vi "RIB Req - MCCB AUX Status.vi"(0 "Limits File Path":path, 5 "Results File Path":path, 11 "error in":errorcluster) -> (4 "Results Data Array":string[][](array[string]), 15 "error out":errorcluster)   [LabVIEW 2024]
doc: "Template test"
uses:
  <vilib>/addons/_JKI Toolkits/State Machine/_JKI_lib_State_Machine.llb/Select State(s)_err__jki_lib_state_machine.vi
  <vilib>/addons/_JKI Toolkits/State Machine/_JKI_lib_State_Machine.llb/Periodic Trigger__ogtk__JKI-SM__jki_lib_state_machine.vi
  <userlib>/_OpenG.lib/file/file.llb/Strip Path Extension - String__ogtk.vi
  <vilib>/Utility/file.llb/Read Delimited Spreadsheet (string).vi
  <userlib>/_OpenG.lib/file/file.llb/openg_file.lvlib
  <userlib>/_OpenG.lib/appcontrol/appcontrol.llb/openg_application_control.lvlib
  <userlib>/_OpenG.lib/time/time.llb/openg_time.lvlib
  <vilib>/Utility/file.llb/Write Delimited Spreadsheet (string).vi
panel:
  in  "UDP Read":string
  in  "connection ID":refnum<k16>
  out "Results Data":string[](array[string])
  in  "handle out":u64
  in  "Exit":bool
  # "Q2 Switch Test"
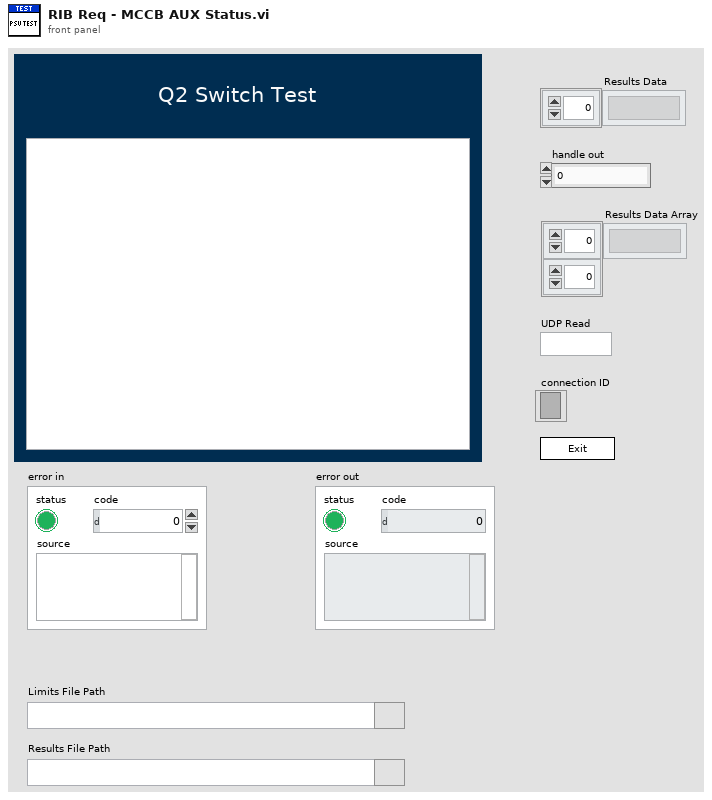
[diagram p1: front panel]
types:
  T1 = enum32{"Invalid", "Standard", "Closed", "Hidden", "Minimized", "Maximized"}
  T2 = enum32{"invalid app kind", "Development System", "Run Time System", "Student Edition", "Embedded LabVIEW", "Evaluation", "Custom"}
  T3 = typedef "FGV - Enum" = enum16{"Cleanup", "Get Data", "Open UDP", "Initialise DAQ", "Initialise I2C"}
  T4 = cluster{"Core":cluster{"Current VI Reference":refnum<vi>, "Close Panel on Exit?":bool}, "Limits File Path":path, "Test Limits":string[][], "Results Data Array":string[][], "Results File Path":path, "Voltage":dbl, "UDP Read":string, "handle out":u64, "connection ID":refnum<k16>}
  T5 = cluster{"Current VI Reference":refnum<vi>, "Close Panel on Exit?":bool}
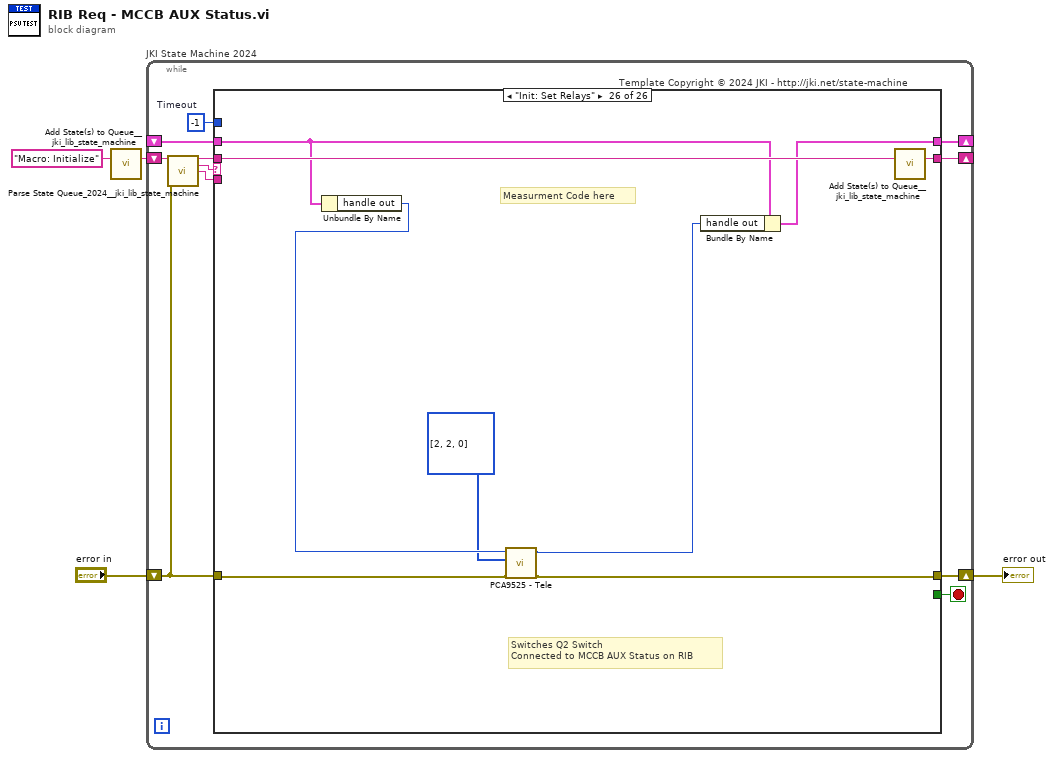
[diagram p0: block diagram]
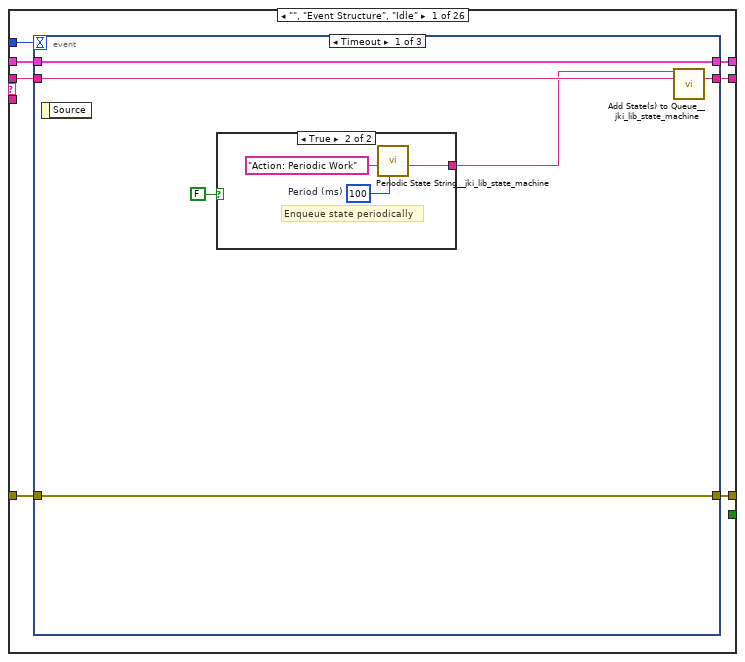
[diagram p2: hidden frame]
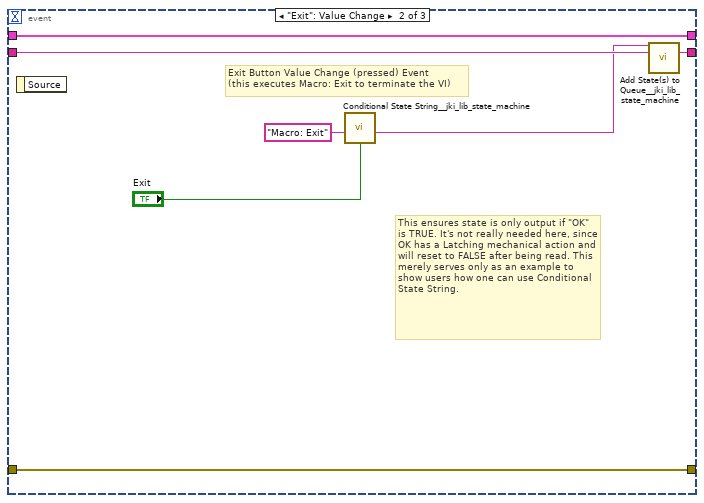
[diagram p4: hidden frame]
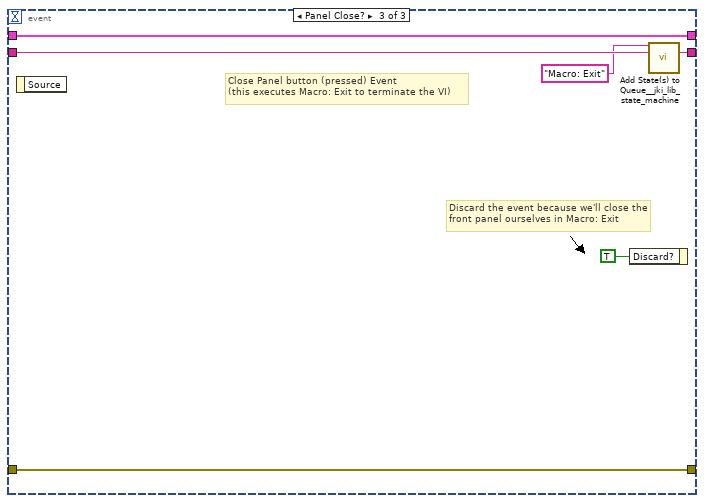
[diagram p5: hidden frame]
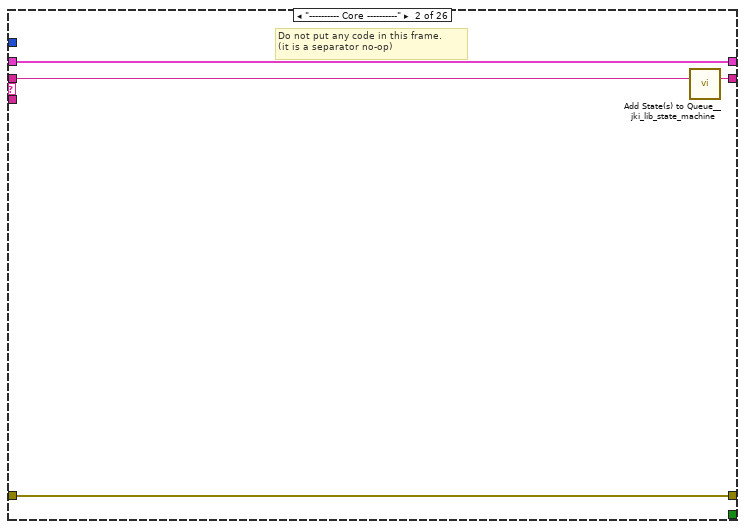
[diagram p6: hidden frame]
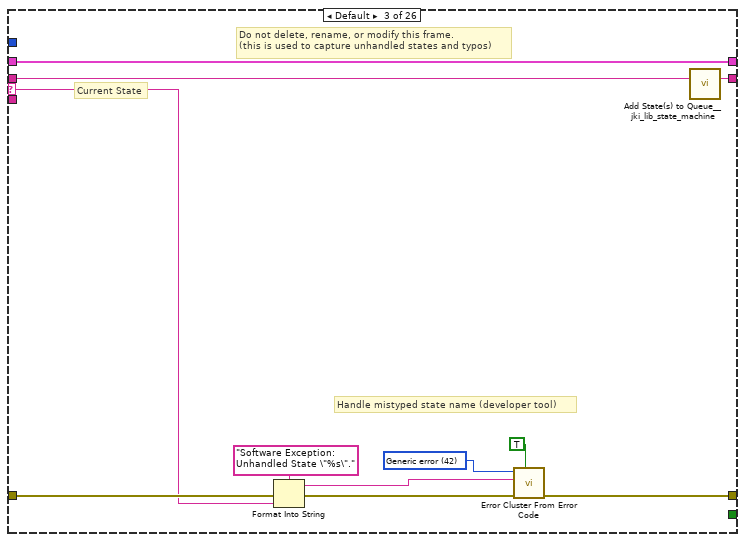
[diagram p7: hidden frame]
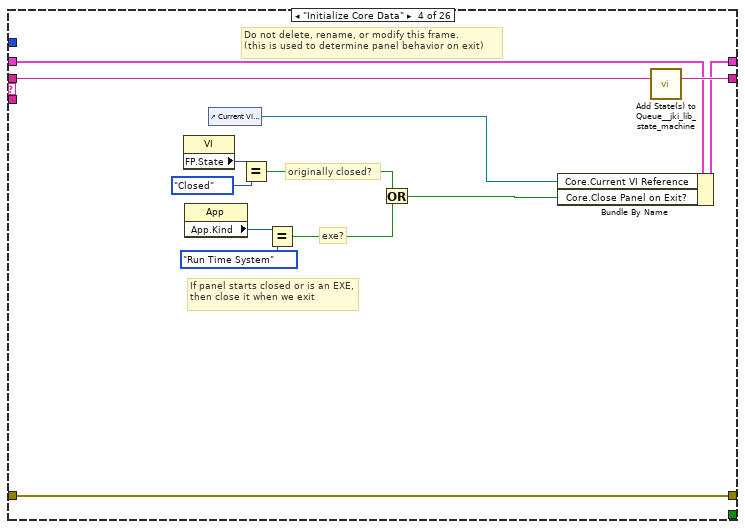
[diagram p8: hidden frame]
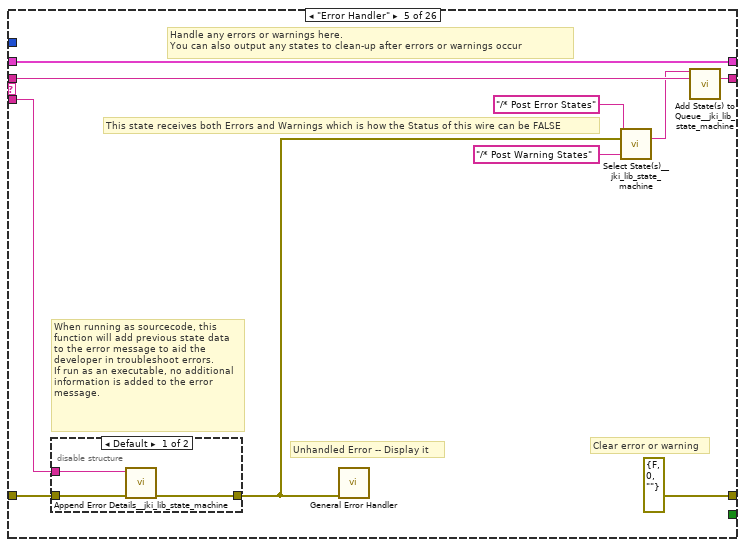
[diagram p9: hidden frame]
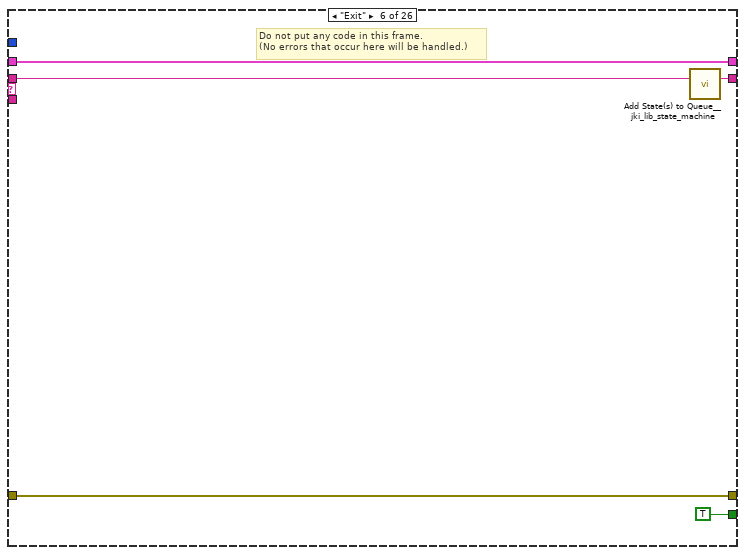
[diagram p11: hidden frame]
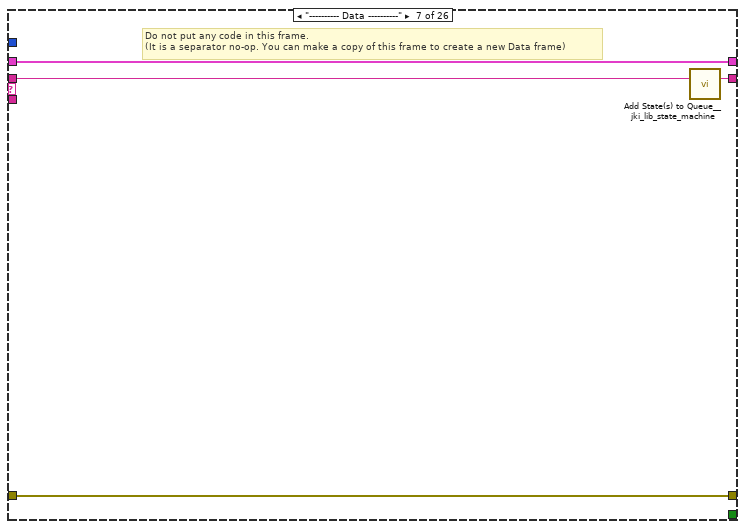
[diagram p12: hidden frame]
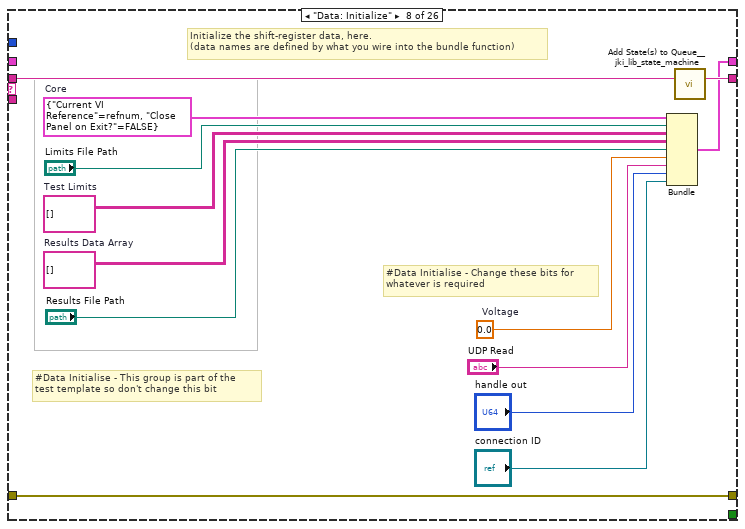
[diagram p13: hidden frame]
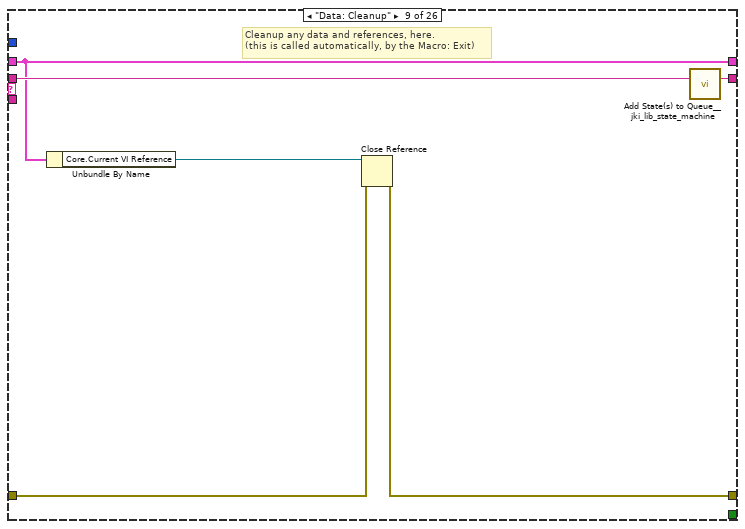
[diagram p14: hidden frame]
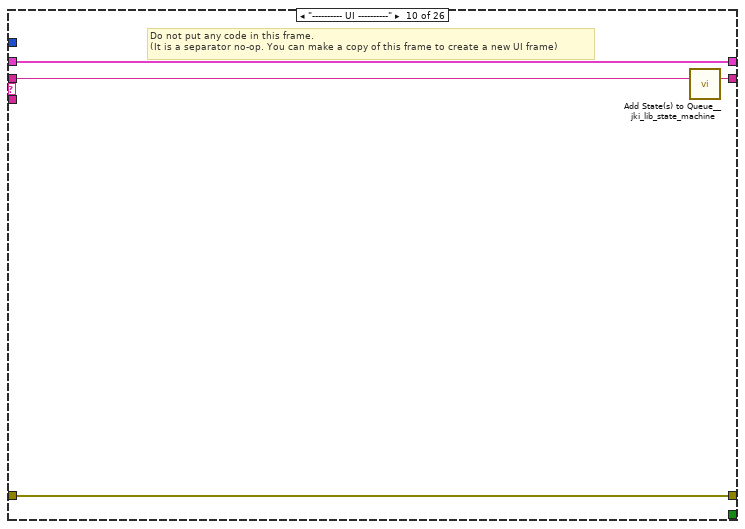
[diagram p15: hidden frame]
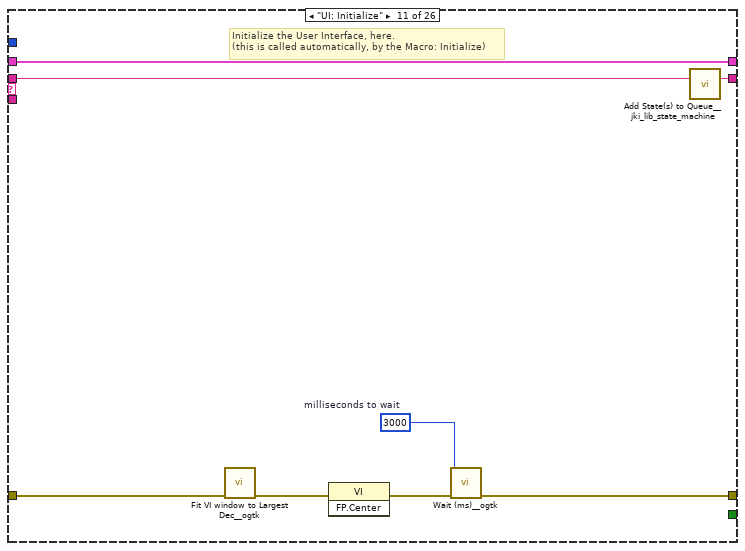
[diagram p16: hidden frame]
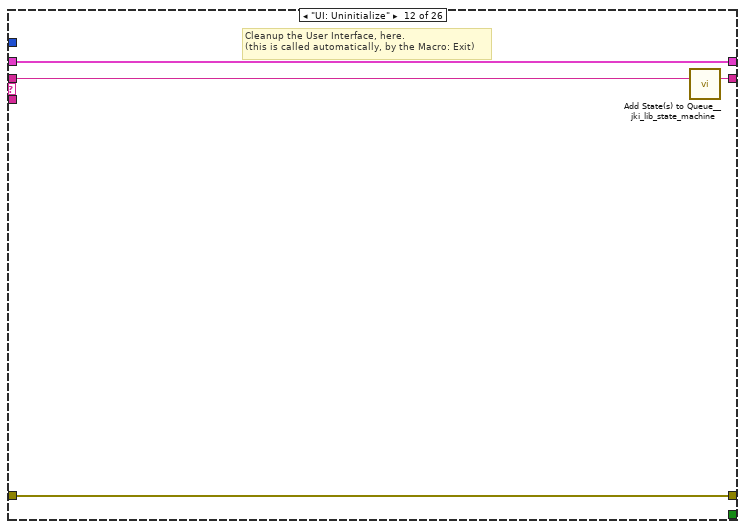
[diagram p17: hidden frame]
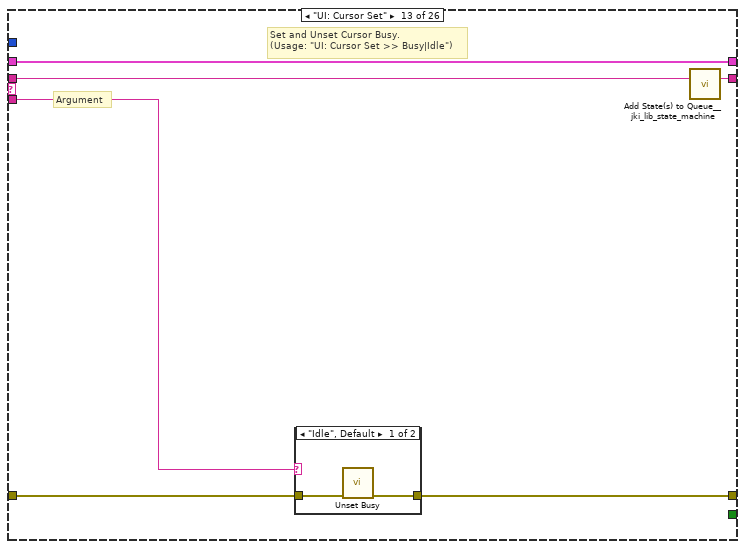
[diagram p18: hidden frame]
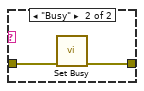
[diagram p19: hidden frame]
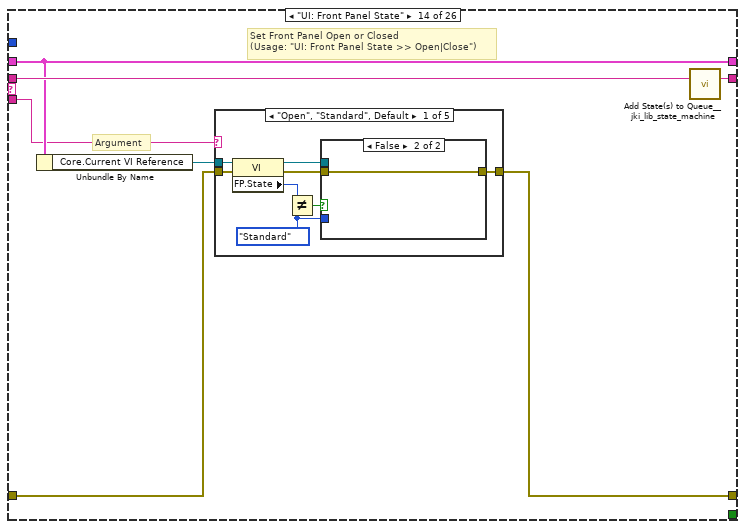
[diagram p20: hidden frame]
diagram:
  n1 = call <vilib>:"Add State(s) to Queue__jki_lib_state_machine.vi"("State(s) in (\"\")"="Macro: Initialize") -> ("States Out"=w4:string)  [unwired: 14 in]
  n2 = while "JKI State Machine 2024" {
    shift-right: [w8] -> _
    shift-left: _ -> [w7]
    shift-right: [w11] -> w1
    shift-left: "error in" -> [w5]
    shift-right: [w10] -> _
    shift-left: w4 -> [w12]
    stop <- w9 stop-if-true
    w6 = -1  # Timeout
    # "Template Copyright © 2024 JKI - http://jki.net/state-machine"
    n3 = call <vilib>:"Parse State Queue_2024__jki_lib_state_machine.vi"("State Queue"=w12, "Error In (no error)"=w5) -> ("Remaining States"=w14:string, "Current State"=w15:string, "Arguments"=w13:string)  [unwired: 11 in]
    n4 = case shown="\"Init: Set Relays\"" w15 {
      selector: w15 -> [_ _ w49 _ _ _ _ _ _ _ _ _ _ _ _ _ _ _ _ _ _ _ _ _ _ _]
      tunnel: w14 -> [w22 w48 w53 w72 w82 w91 w95 w108 w114 w118 w126 w130 w136 w147 w216 w221 w226 w235 w239 w252 w269 w273 w282 w286 w294 w303]
      tunnel: w13 -> [_ _ _ _ w77 _ _ _ _ _ _ _ w131 w141 _ _ _ _ _ _ _ _ _ _ _ _]
      tunnel: w7 -> [w20 w45 w51 w65 w79 w89 w92 _ w109 w115 w124 w128 w134 w143 w213 w218 w223 w233 w236 w242 w261 w270 w278 w283 w292 w300]
      tunnel: [w19 w46 w55 w69 errorcluster {"status"=FALSE, "code"=0, "source"=""} ("error out") w88 w93 w105 w110 w116 w122 w127 w132 w144 w214 w219 w224 w230 w237 w248 w266 w271 w280 w284 w289 w298] -> w11
      tunnel: w5 -> [w16 w46 w54 w69 w78 w88 w93 w105 w111 w116 w123 w127 w133 w145 w214 w219 w224 w230 w237 w247 w265 w271 w279 w284 w290 w299]
      tunnel: [w21 w47 w52 w71 w81 w90 w94 w107 w113 w117 w125 w129 w135 w146 w215 w220 w225 w234 w238 w251 w268 w272 w281 w285 w293 w302] -> w10
      tunnel: [_ _ _ _ _ TRUE _ _ _ _ _ _ _ _ _ _ _ _ _ _ _ _ _ _ _ _] -> w9
      tunnel: [w18 w45 w51 w70 w79 w89 w92 w106 w109 w115 w124 w128 w134 w143 w213 w218 w223 w233 w236 w241 w260 w270 w278 w283 w291 w301] -> w8
      tunnel: w6 -> [w17 _ _ _ _ _ _ _ _ _ _ _ _ _ _ _ _ _ _ _ _ _ _ _ _ _]
      frame "", "Event Structure", "Idle" {
        n5 = event shown="[0] Timeout" {
          selector: _ -> [_ _ _]
          dyn-events: _ -> [_ _ _]
          timeout: w17 -> [_ _ _]
          tunnel: w22 -> [w28 w38 w44]
          tunnel: [w27 w37 w43] -> w21
          tunnel: w20 -> [w25 w35 w41]
          tunnel: [w26 w36 w42] -> w19
          tunnel: w16 -> [w26 w36 w42]
          tunnel: [w25 w35 w41] -> w18
          event Timeout {
            n6 = event-data() -> ()  [unwired: 1 in, 1 out]
            n7 = case shown="True" FALSE {
              tunnel: [_ w31] -> w24
              frame False {
              }
              frame True {
                w29 = u32 100  # Period (ms)
                # "Enqueue state periodically"
                n8 = call <vilib>:"Periodic State String__jki_lib_state_machine.vi"("Period (ms)"=w29, "State"="Action: Periodic Work") -> ("State Out"=w31:string)  [unwired: 9 in]
              }
            }
            n9 = call <vilib>:"Add State(s) to Queue__jki_lib_state_machine.vi"("State(s) in Front (\"\")"=w24, "State(s) in (\"\")"=w28) -> ("States Out"=w27:string)  [unwired: 13 in]
          }
          event "Exit": Value Change {
            # "This ensures state is only output if \"OK\" is TRUE. It's not really needed here, since OK has a Latching mechanical action and will reset to FALSE after being read. This merely serves only as an example to show users how one can use Conditional State String."
            # "Exit Button Value Change (pressed) Event\n(this executes Macro: Exit to terminate the VI)"
            n10 = event-data() -> ()  [unwired: 1 in, 1 out]
            n11 = call <vilib>:"Conditional State String__jki_lib_state_machine.vi"("Do State(s)?"="Exit", "State"="Macro: Exit") -> ("State Out"=w32:string)  [unwired: 7 in]
            n12 = call <vilib>:"Add State(s) to Queue__jki_lib_state_machine.vi"("State(s) in Front (\"\")"=w32, "State(s) in (\"\")"=w38) -> ("States Out"=w37:string)  [unwired: 13 in]
          }
          event Panel Close? {
            # "Discard the event because we'll close the front panel ourselves in Macro: Exit"
            # "Close Panel button (pressed) Event\n(this executes Macro: Exit to terminate the VI)"
            n13 = event-data() -> ()  [unwired: 1 in, 1 out]
            n14 = event-data("Discard?"=TRUE) -> ()  [unwired: 1 in, 1 out]
            n15 = call <vilib>:"Add State(s) to Queue__jki_lib_state_machine.vi"("State(s) in Front (\"\")"="Macro: Exit", "State(s) in (\"\")"=w44) -> ("States Out"=w43:string)  [unwired: 13 in]
          }
        }
      }
      frame "---------- Core ----------" {
        # "Do not put any code in this frame.\n(it is a separator no-op)"
        n16 = call <vilib>:"Add State(s) to Queue__jki_lib_state_machine.vi"("State(s) in (\"\")"=w48) -> ("States Out"=w47:string)  [unwired: 14 in]
      }
      frame Default {
        w58 = 42 items=["No error", "Argument error", "Memory is full", "Out of zone", "End of file", "File already open", "Generic file I/O error", "File not found", "File permission error", "Disk is full", "Duplicate path", "Too many files open", "System feature not enabled", "Resource file not found", "Cannot add resource", "Resource not found", "Image not found", "Image memory error", "Pen does not exist", "Config type invalid", "Config token not found", "Config parse error", "Config memory error", "Bad external code format", "Bad external code offset", "External code not present", "Null window", "Destroy window error", "Null menu", "Print aborted", "Bad print record", "Print driver error", "Windows error during printing", "Memory error during printing", "Print dialog error", "Generic print error", "Invalid device refnum", "Device not found", "Device parameter error", "Device unit error", "Cannot open device", "Device call aborted", "Generic error", "Cancelled by user", "Object ID too low", "Object ID too high", "Object not in heap", "Unknown heap", "Unknown object (invalid DefProc)", "Unknown object (DefProc not in table)", "Message out of range", "Invalid (null) method", "Unknown message", "Manager call not supported", "Bad address", "Network operation in progress", "Network operation timed out", "Connection is busy", "Network attribute not supported", "Network error", "Address in use", "System out of memory", "Connection aborted", "Connection refused", "Not connected", "Already connected", "Connection closed", "Initialization error (interapplication manager)", "Bad occurrence", "Wait on unbound occurrence handler", "Occurrence queue overflow", "Datalog type conflict", "Unused", "Unrecognized type (interapplication manager)", "Memory corrupt", "Failed to make temporary DLL", "Old CIN version", "Drag socket not found", "Failed to load drop-object", "Failed to register OLE object", "Failed to release OLE object", "Format specifier type mismatch", "Unknown format specifier", "Too few format specifiers", "Too many format specifiers", "Scan failed", "Newer CIN version", "Error converting to variant", "Runtime menu error", "Password tampered", "Variant attribute not found", "Incompatible variant data type", "Event data is not available", "Event Store is not present", "Occurrence is not found", "Event Queue is not created", "Event info is not available", "Refnum passed is NULL", "Error retrieving Class GUID", "Error retrieving CoClass GUID", "Error retrieving TypeLib GUID.", "Bad built application magic bytes.", "Specific driver is different from the specific driver associated with the Logical Name.", "There is no session opened to the class driver.", "Max Error", "MAX - Error with config objects", "MAX - Error loading configuration", "MAX - Group not supported"]
        # "Current State"
        # "Do not delete, rename, or modify this frame.\n(this is used to capture unhandled states and typos)"
        # "Handle mistyped state name (developer tool)"
        n17 = Format Into String(format string="Software Exception: Unhandled State \"%s\"." ("message"), error in=w54, w49) -> (resulting string=w57:string, error out=w56:errorcluster)  [unwired: 1 in]
        n18 = call <vilib>:"Error Cluster From Error Code.vi"("show call chain? (False)"=TRUE, "error in (no error)"=w56, "error message (\"\")"=w57, "error code (0)"=w58) -> ("error out"=w55:errorcluster)  [unwired: 5 in]
        n19 = call <vilib>:"Add State(s) to Queue__jki_lib_state_machine.vi"("State(s) in (\"\")"=w53) -> ("States Out"=w52:string)  [unwired: 14 in]
      }
      frame "Initialize Core Data" {
        # "Do not delete, rename, or modify this frame.\n(this is used to determine panel behavior on exit)"
        # "originally closed?"
        # "exe?"
        # "If panel starts closed or is an EXE, then close it when we exit"
        n20 = property class="VI"() -> ("FP.State"=w62:T1)  [unwired: 2 in, 2 out]
        n21 = property class="App"() -> ("App.Kind"=w68:T2)  [unwired: 2 in, 2 out]
        n22 = control-ref of="Current VI Reference"() -> (w63:refnum<vi>)
        n23 = Equal?(x=w62, y=T1."Closed" ("Front Panel Window:State")) -> (x = y?=w60:bool)
        n24 = Equal?(x=w68, y=T2."Run Time System" ("Application:Kind")) -> (x = y?=w66:bool)
        n25 = Or(x=w60, y=w66) -> (x .or. y?=w64:bool)
        n26 = Bundle By Name(cluster=w65, "Core.Current VI Reference"=w63, "Core.Close Panel on Exit?"=w64) -> (w70:T4)
        n27 = call <vilib>:"Add State(s) to Queue__jki_lib_state_machine.vi"("State(s) in (\"\")"=w72) -> ("States Out"=w71:string)  [unwired: 14 in]
      }
      frame "Error Handler" {
        # "When running as sourcecode, this function will add previous state data to the error message to aid the developer in troubleshoot errors.\nIf run as an executable, no additional information is added to the error message."
        # "This state receives both Errors and Warnings which is how the Status of this wire can be FALSE"
        # "Unhandled Error -- Display it"
        # "Handle any errors or warnings here.\nYou can also output any states to clean-up after errors or warnings occur"
        # "Clear error or warning"
        n28 = disable-structure shown="Default" {
          disable-tunnel: w78 -> [w85 w86]
          disable-tunnel: w77 -> [w84 _]
          disable-tunnel: [w83 w86] -> w76
          frame condition #0 (active) {
            n29 = call <vilib>:"Append Error Details__jki_lib_state_machine.vi"("error in (no error)"=w85, "Previous State and Argument(s)"=w84) -> ("error out"=w83:errorcluster)  [unwired: 9 in]
          }
          frame condition #1 {
          }
        }
        n30 = call <vilib>:"General Error Handler.vi"("error in (no error)"=w76) -> ()  [unwired: 10 in, 5 out]
        n31 = call-poly <vilib>:"Select State(s)__jki_lib_state_machine.vi"("State(s) if True (\"\")"="/* Post Error States", "Select"=w76, "State(s) if False (\"\")"="/* Post Warning States") -> ("States Out"=w74:string)  [unwired: 12 in]
        n32 = call <vilib>:"Add State(s) to Queue__jki_lib_state_machine.vi"("State(s) in Front (\"\")"=w74, "State(s) in (\"\")"=w82) -> ("States Out"=w81:string)  [unwired: 13 in]
      }
      frame "Exit" {
        # "Do not put any code in this frame.\n(No errors that occur here will be handled.)"
        n33 = call <vilib>:"Add State(s) to Queue__jki_lib_state_machine.vi"("State(s) in (\"\")"=w91) -> ("States Out"=w90:string)  [unwired: 14 in]
      }
      frame "---------- Data ----------" {
        # "Do not put any code in this frame.\n(It is a separator no-op. You can make a copy of this frame to create a new Data frame)"
        n34 = call <vilib>:"Add State(s) to Queue__jki_lib_state_machine.vi"("State(s) in (\"\")"=w95) -> ("States Out"=w94:string)  [unwired: 14 in]
      }
      frame "Data: Initialize" {
        w99 = 0.0  # Voltage
        w101 = string[][] []  # Results Data Array
        w102 = string[][] []  # Test Limits
        w104 = T5 {"Current VI Reference"=refnum, "Close Panel on Exit?"=FALSE}  # Core
        # "#Data Initialise - Change these bits for\nwhatever is required"
        # "#Data Initialise - This group is part of the\ntest template so don't change this bit"
        # "Initialize the shift-register data, here.\n(data names are defined by what you wire into the bundle function)"
        n35 = Bundle("Core"=w104, "Limits File Path"="Limits File Path", "Test Limits"=w102, "Results Data Array"=w101, "Results File Path"="Results File Path", "Voltage"=w99, "UDP Read"="UDP Read", "handle out"="handle out", "connection ID"="connection ID") -> (w106:T4)  [unwired: 1 in]
        n36 = call <vilib>:"Add State(s) to Queue__jki_lib_state_machine.vi"("State(s) in (\"\")"=w108) -> ("States Out"=w107:string)  [unwired: 14 in]
      }
      frame "Data: Cleanup" {
        # "Cleanup any data and references, here.\n(this is called automatically, by the Macro: Exit)"
        n37 = Unbundle By Name(w109) -> ("Core.Current VI Reference"=w112:refnum<vi>)
        n38 = Close Reference(reference=w112, error in (no error)=w111) -> (error out=w110:errorcluster)
        n39 = call <vilib>:"Add State(s) to Queue__jki_lib_state_machine.vi"("State(s) in (\"\")"=w114) -> ("States Out"=w113:string)  [unwired: 14 in]
      }
      frame "---------- UI ----------" {
        # "Do not put any code in this frame.\n(It is a separator no-op. You can make a copy of this frame to create a new UI frame)"
        n40 = call <vilib>:"Add State(s) to Queue__jki_lib_state_machine.vi"("State(s) in (\"\")"=w118) -> ("States Out"=w117:string)  [unwired: 14 in]
      }
      frame "UI: Initialize" {
        w121 = u32 3000  # milliseconds to wait
        # "Initialize the User Interface, here.\n(this is called automatically, by the Macro: Initialize)"
        n41 = call <userlib>:"Fit VI window to Largest Dec__ogtk.vi"("error in (no error)"=w123) -> ("error out"=w119:errorcluster)  [unwired: 5 in, 1 out]
        n42 = invoke class="VI" method="FP.Center"(error in=w119) -> (error out=w120:errorcluster)  [unwired: 2 in, 2 out]
        n43 = call <userlib>:"Wait (ms)__ogtk.vi"("error in (no error)"=w120, "milliseconds to wait"=w121) -> ("error out"=w122:errorcluster)  [unwired: 8 in, 1 out]
        n44 = call <vilib>:"Add State(s) to Queue__jki_lib_state_machine.vi"("State(s) in (\"\")"=w126) -> ("States Out"=w125:string)  [unwired: 14 in]
      }
      frame "UI: Uninitialize" {
        # "Cleanup the User Interface, here.\n(this is called automatically, by the Macro: Exit)"
        n45 = call <vilib>:"Add State(s) to Queue__jki_lib_state_machine.vi"("State(s) in (\"\")"=w130) -> ("States Out"=w129:string)  [unwired: 14 in]
      }
      frame "UI: Cursor Set" {
        # "Argument"
        # "Set and Unset Cursor Busy.\n(Usage: \"UI: Cursor Set >> Busy|Idle\")"
        n46 = case shown="\"Idle\", Default" w131 {
          tunnel: w133 -> [w138 w140]
          tunnel: [w137 w139] -> w132
          frame "Idle", Default {
            n47 = call <vilib>:"Unset Busy.vi"("error in (no error)"=w138) -> ("error out"=w137:errorcluster)  [unwired: 10 in]
          }
          frame "Busy" {
            n48 = call <vilib>:"Set Busy.vi"("error in (no error)"=w140) -> ("error out"=w139:errorcluster)  [unwired: 9 in, 1 out]
          }
        }
        n49 = call <vilib>:"Add State(s) to Queue__jki_lib_state_machine.vi"("State(s) in (\"\")"=w136) -> ("States Out"=w135:string)  [unwired: 14 in]
      }
      frame "UI: Front Panel State" {
        # "Argument"
        # "Set Front Panel Open or Closed\n(Usage: \"UI: Front Panel State >> Open|Close\")"
        n50 = Unbundle By Name(w143) -> ("Core.Current VI Reference"=w142:refnum<vi>)
        n51 = case shown="\"Open\", \"Standard\", Default" w141 {
          tunnel: w145 -> [w153 w168 w179 w192 w205]
          tunnel: [w155 w169 w181 w194 w207] -> w144
          tunnel: w142 -> [w154 w166 w180 w193 w206]
          frame "Open", "Standard", Default {
            w148 = T1."Standard" ("State")
            n52 = property class="VI"(reference=w154, error in=w153) -> (reference out=w151:refnum<vi>, error out=w152:errorcluster, "FP.State"=w150:T1)
            n53 = Not Equal?(x=w150, y=w148) -> (x != y?=w149:bool)
            n54 = case shown="False" w149 {
              tunnel: [w159 w161] -> w155
              tunnel: w152 -> [w158 w161]
              tunnel: w151 -> [w157 _]
              tunnel: w148 -> [w156 _]
              frame True {
                n55 = invoke class="VI" method="FP.Open"(reference=w157, error in=w158, "Activate"=TRUE, "State"=w156) -> (error out=w159:errorcluster)  [unwired: 1 in, 4 out]
              }
              frame False {
              }
            }
          }
          frame "Close", "Closed" {
            n56 = property class="VI"(reference=w166, error in=w168) -> (reference out=w165:refnum<vi>, error out=w167:errorcluster, "FP.State"=w163:T1)
            n57 = Not Equal?(x=w163, y=T1."Closed" ("Front Panel Window:State")) -> (x != y?=w162:bool)
            n58 = case shown="True" w162 {
              tunnel: [w170 w173] -> w169
              tunnel: w167 -> [w170 w172]
              tunnel: w165 -> [_ w171]
              frame False {
              }
              frame True {
                n59 = invoke class="VI" method="FP.Close"(reference=w171, error in=w172) -> (error out=w173:errorcluster)  [unwired: 1 in, 2 out]
              }
            }
          }
          frame "Hidden", "Hide" {
            w174 = T1."Hidden" ("State")
            n60 = property class="VI"(reference=w180, error in=w179) -> (reference out=w177:refnum<vi>, error out=w178:errorcluster, "FP.State"=w176:T1)
            n61 = Not Equal?(x=w176, y=w174) -> (x != y?=w175:bool)
            n62 = case shown="True" w175 {
              tunnel: [w185 w186] -> w181
              tunnel: w178 -> [w184 w186]
              tunnel: w177 -> [w183 _]
              tunnel: w174 -> [w182 _]
              frame True {
                n63 = invoke class="VI" method="FP.Open"(reference=w183, error in=w184, "State"=w182) -> (error out=w185:errorcluster)  [unwired: 2 in, 4 out]
              }
              frame False {
              }
            }
          }
          frame "Minimize", "Minimized" {
            w187 = T1."Minimized" ("State")
            n64 = property class="VI"(reference=w193, error in=w192) -> (reference out=w190:refnum<vi>, error out=w191:errorcluster, "FP.State"=w189:T1)
            n65 = Not Equal?(x=w189, y=w187) -> (x != y?=w188:bool)
            n66 = case shown="True" w188 {
              tunnel: [w198 w199] -> w194
              tunnel: w191 -> [w197 w199]
              tunnel: w190 -> [w196 _]
              tunnel: w187 -> [w195 _]
              frame True {
                n67 = invoke class="VI" method="FP.Open"(reference=w196, error in=w197, "State"=w195) -> (error out=w198:errorcluster)  [unwired: 2 in, 4 out]
              }
              frame False {
              }
            }
          }
          frame "Maximize", "Maximized" {
            w200 = T1."Maximized" ("State")
            n68 = property class="VI"(reference=w206, error in=w205) -> (reference out=w203:refnum<vi>, error out=w204:errorcluster, "FP.State"=w202:T1)
            n69 = Not Equal?(x=w202, y=w200) -> (x != y?=w201:bool)
            n70 = case shown="True" w201 {
              tunnel: [w211 w212] -> w207
              tunnel: w204 -> [w210 w212]
              tunnel: w203 -> [w209 _]
              tunnel: w200 -> [w208 _]
              frame True {
                n71 = invoke class="VI" method="FP.Open"(reference=w209, error in=w210, "State"=w208) -> (error out=w211:errorcluster)  [unwired: 2 in, 4 out]
              }
              frame False {
              }
            }
          }
        }
        n72 = call <vilib>:"Add State(s) to Queue__jki_lib_state_machine.vi"("State(s) in (\"\")"=w147) -> ("States Out"=w146:string)  [unwired: 14 in]
      }
      frame "---------- Macro ----------" {
        # "Do not put any code in this frame.\n(It is a separator no-op. You can make a copy of this frame to create a new Macro frame)"
        n73 = call <vilib>:"Add State(s) to Queue__jki_lib_state_machine.vi"("State(s) in (\"\")"=w216) -> ("States Out"=w215:string)  [unwired: 14 in]
      }
      frame "Macro: Initialize" {
        # "Initialization Macro\n(This is called once, when the VI starts)"
        n74 = call <vilib>:"Add State(s) to Queue__jki_lib_state_machine.vi"("State(s) in Front (\"\")"="Data: Initialize\nInitialize Core Data\nUI: Initialize\nUI: Front Panel State >> Open\nInit: Initialise\nMacro: Test", "State(s) in (\"\")"=w221) -> ("States Out"=w220:string)  [unwired: 13 in]
      }
      frame "Macro: Test" {
        # "#Test Macro - Add the sequence \nfor measurments and limits testing here"
        n75 = call <vilib>:"Add State(s) to Queue__jki_lib_state_machine.vi"("State(s) in Front (\"\")"="Limits Test: Read Limits File\nInit: Set Relays\nLimits Test: Handle Out Test\nResults Data: Write Results Data\nMacro: Exit", "State(s) in (\"\")"=w226) -> ("States Out"=w225:string)  [unwired: 13 in]
      }
      frame "Macro: Exit" {
        # "Exit Macro\n(This is called once, when the VI exits)"
        n76 = Unbundle By Name(w233) -> ("Core.Close Panel on Exit?"=w228:bool)
        n77 = call <vilib>:"Conditional State String__jki_lib_state_machine.vi"("Do State(s)?"=w228, "State"="UI: Front Panel State >> Close") -> ("State Out"=w227:string)  [unwired: 7 in]
        n78 = call <vilib>:"Add State(s) to Queue__jki_lib_state_machine.vi"("State(s) in (\"\")"=w227, "State(s) at Back (\"\")"="UI: Uninitialize\nData: Cleanup\nExit") -> ("States Out"=w231:string)  [unwired: 13 in]
        n79 = call <vilib>:"Add State(s) to Queue__jki_lib_state_machine.vi"("State(s) in Front (\"\")"=w231, "State(s) in (\"\")"=w235) -> ("States Out"=w234:string)  [unwired: 13 in]
      }
      frame "---------- Limits Test ----------" {
        # "Template Separator\n(You can make a copy of, or modify, this frame)"
        n80 = call <vilib>:"Add State(s) to Queue__jki_lib_state_machine.vi"("State(s) in (\"\")"=w239) -> ("States Out"=w238:string)  [unwired: 14 in]
      }
      frame "Limits Test: Read Limits File" {
        w245 = ","  # delimiter (\t)
        n81 = Unbundle By Name(w242) -> ("Limits File Path"=w246:path)
        n82 = Current VI's Path "Test Case Path"() -> (path=w250:path)
        n83 = call-poly <vilib>:"Read Delimited Spreadsheet.vi"("file path (dialog if empty)"=w246, "error in (no error)"=w247, "delimiter (\\t)"=w245) -> ("all rows"=w243:string[][], "error out"=w248:errorcluster)  [unwired: 7 in, 4 out]
        n84 = Strip Path(path=w250) -> (name=w249:string)  [unwired: 1 out]
        n85 = call-poly <userlib>:"Strip Path Extension__ogtk.vi"("path"=w249) -> ("root"=w244:string)  [unwired: 1 out]
        n86 = for {
          tunnel: w244 -> [w256]
          tunnel: w243 -> [w254] mode=indexing
          tunnel: [w254] -> w240 mode=indexing if=w253
          n87 = Index Array(array=w254) -> (element=w255:string)  [unwired: 1 in]
          n88 = Equal?(x=w256, y=w255) -> (x = y?=w253:bool)
        }
        n89 = Bundle By Name(cluster=w242, "Test Limits"=w240) -> (w241:T4)
        n90 = call <vilib>:"Add State(s) to Queue__jki_lib_state_machine.vi"("State(s) in (\"\")"=w252) -> ("States Out"=w251:string)  [unwired: 14 in]
      }
      frame "Limits Test: Handle Out Test" {
        w262 = "Handle Out Test"  # Sub Test Name
        # "Handle Out Test = Equal 0 = Fail\nHandle Out Test = Not Equal 0 = Pass"
        # "#Limits Testing - Add the sub test name for\ntest included in limits file"
        n91 = Unbundle By Name(w261) -> ("Results Data Array"=w259:string[][])
        n92 = Unbundle By Name(w261) -> ("Test Limits"=w263:string[][], "handle out"=w267:u64)
        n93 = To Variant(anything=w267) -> (Variant=w264:variant)
        n94 = call "Process Results.vi"("error in (no error)"=w265, "Measurement"=w264, "Test Limits"=w263, "Sub Test Name"=w262) -> ("error out"=w266:errorcluster, "Results Data"=w257:string[])  [unwired: 6 in]
        "Results Data" <- w257
        n95 = Build Array (concatenate)(w259, w257) -> (w258:string[][])
        n96 = Bundle By Name(cluster=w261, "Results Data Array"=w258) -> (w260:T4)
        n97 = call <vilib>:"Add State(s) to Queue__jki_lib_state_machine.vi"("State(s) in (\"\")"=w269) -> ("States Out"=w268:string)  [unwired: 14 in]
      }
      frame "---------- Results Data ----------" {
        # "Template Separator\n(You can make a copy of, or modify, this frame)"
        n98 = call <vilib>:"Add State(s) to Queue__jki_lib_state_machine.vi"("State(s) in (\"\")"=w273) -> ("States Out"=w272:string)  [unwired: 14 in]
      }
      frame "Results Data: Write Results Data" {
        w275 = ","  # delimiter (\t)
        w276 = TRUE  # append to file? (new file:F)
        n99 = Unbundle By Name(w278) -> ("Results File Path"=w277:path, "Results Data Array"=w274:string[][])
        "Results Data Array" <- w274
        n100 = call-poly <vilib>:"Write Delimited Spreadsheet.vi"("file path (dialog if empty)"=w277, "2D data"=w274, "append to file? (new file:F)"=w276, "error in (no error)"=w279, "delimiter (\\t)"=w275) -> ("error out"=w280:errorcluster)  [unwired: 9 in, 1 out]
        n101 = call <vilib>:"Add State(s) to Queue__jki_lib_state_machine.vi"("State(s) in (\"\")"=w282) -> ("States Out"=w281:string)  [unwired: 14 in]
      }
      frame "---------- Init ----------" {
        # "Template Separator\n(You can make a copy of, or modify, this frame)"
        n102 = call <vilib>:"Add State(s) to Queue__jki_lib_state_machine.vi"("State(s) in (\"\")"=w286) -> ("States Out"=w285:string)  [unwired: 14 in]
      }
      frame "Init: Initialise" {
        # "Measurement initialisation code goes here"
        n103 = call "FGV - Initialise.vi"("Enum"=FGV_-_Enum."Get Data", "Error In"=w290) -> ("Handle Out"=w287:u64, "Error Out"=w289:errorcluster)  [unwired: 10 in, 2 out]
        n104 = Bundle By Name(cluster=w292, "handle out"=w287) -> (w291:T4)
        n105 = call <vilib>:"Add State(s) to Queue__jki_lib_state_machine.vi"("State(s) in (\"\")"=w294) -> ("States Out"=w293:string)  [unwired: 14 in]
      }
      frame "Init: Set Relays" {
        # "Switches Q2 Switch\nConnected to MCCB AUX Status on RIB"
        # "Measurment Code here"
        n106 = Unbundle By Name(w300) -> ("handle out"=w296:u64)
        n107 = call "PCA9525 - Tele.vi"("error in (no error)"=w299, "buffer"=u8[] [2, 2, 0], "handle"=w296) -> ("error out"=w298:errorcluster, "handle out"=w297:u64)  [unwired: 6 in, 1 out]
        n108 = Bundle By Name(cluster=w300, "handle out"=w297) -> (w301:T4)
        n109 = call <vilib>:"Add State(s) to Queue__jki_lib_state_machine.vi"("State(s) in (\"\")"=w303) -> ("States Out"=w302:string)  [unwired: 14 in]
      }
    }
  }
  "error out" <- w1
